vi "obtain_queue.vi"(8 "error in (no error)":errorcluster) -> (0 "error out":errorcluster, 3 "queue out":refnum<queue>)   [LabVIEW 2020]
uses:
  message.ctl
  states.ctl
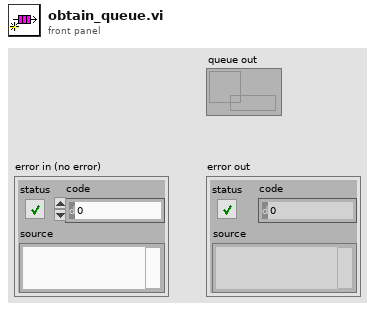
[diagram p1: front panel]
types:
  T1 = typedef "message.ctl" = cluster{"states":T2, "Payload":variant}
  T2 = typedef "states.ctl" = enum16{"update temperature (API)", "update temperature (User)", "stop"}
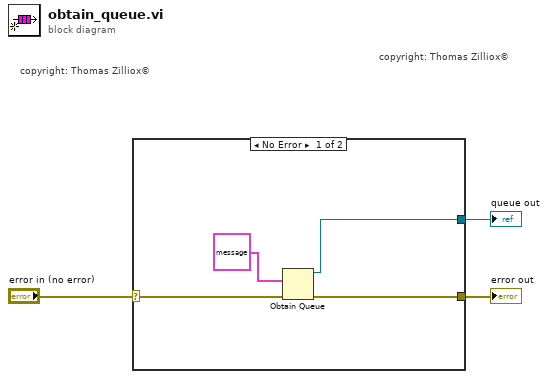
[diagram p0: block diagram]
diagram:
  # "copyright: Thomas Zilliox©"
  # "copyright: Thomas Zilliox©"
  n1 = case shown="No Error" "error in (no error)" {
    selector: "error in (no error)" -> [w7 w8]
    tunnel: [w6 w8] -> w2
    tunnel: [w4 _] -> w1
    frame No Error {
      n2 = Obtain Queue(element data type=T1 {"states"=enum."update temperature (API)", "Payload"=variant} ("Message"), error in (no error)=w7) -> (queue out=w4:refnum<queue>, error out=w6:errorcluster)  [unwired: 3 in, 1 out]
    }
    frame Error {
    }
  }
  "error out" <- w2
  "queue out" <- w1
